vi "get_status.vi"(8 "error in":errorcluster, 11 "VISA resource name in":refnum<visa-resource-name>="COM1") -> (0 "error out":errorcluster, 2 "status":string, 3 "VISA resource name out":refnum<visa-resource-name>)   [LabVIEW 2020]
panel:
  in  "Read count":u32
  out "command":string
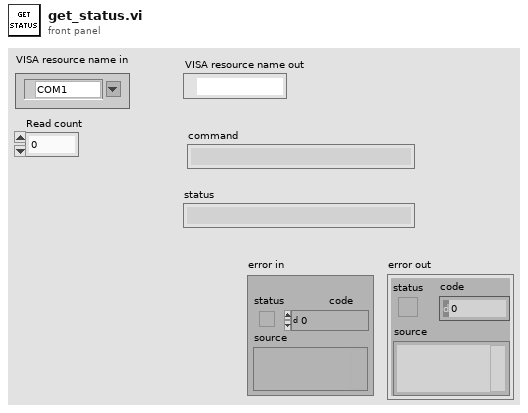
[diagram p1: front panel]
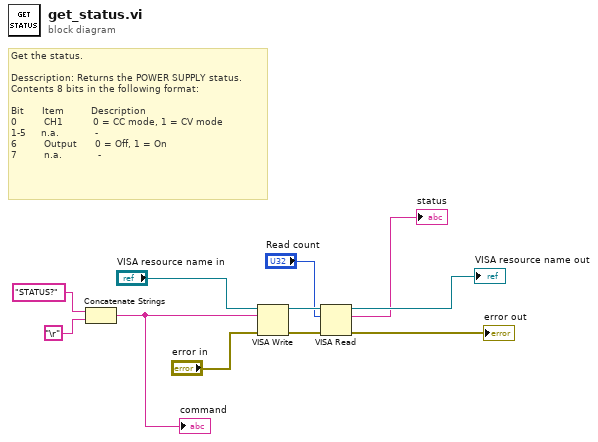
[diagram p0: block diagram]
diagram:
  # "Get the status.\n\nDesscription: Returns the POWER SUPPLY status.\nContents 8 bits in the following format:\n\nBit      Item         Description\n0         CH1          0 = CC mode, 1 = CV mode\n1-5     n.a.            -\n6         Output      0 = Off, 1 = On\n7         n.a.            -"
  n1 = Concatenate Strings("STATUS?" ("string"), "\r") -> (w8:string)
  "command" <- w8
  n2 = VISA Write(VISA resource name="VISA resource name in", write buffer=w8, error in (no error)="error in") -> (VISA resource name out=w6:refnum<visa-resource-name>, error out=w5:errorcluster)  [unwired: 1 out]
  n3 = VISA Read(VISA resource name=w6, byte count="Read count", error in (no error)=w5) -> (VISA resource name out=→"VISA resource name out":refnum<visa-resource-name>, read buffer=→"status":string, error out=→"error out":errorcluster)  [unwired: 1 out]
